vi "Read Refs.vi"(11 "Base Actor in":refnum<class "Base Actor.lvclass">) -> (2 "Refs":refnum<class "Refs.lvclass">)   [LabVIEW 2020, in "jettl.lvlib" / "Base jettl Actor.lvlib" / "Base Actor.lvlib" / "Base Actor.lvclass"]
uses:
  Base Actor.lvclass
  Refs/Refs.lvclass
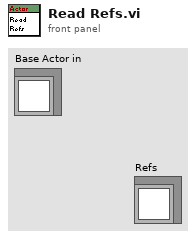
[diagram p1: front panel]
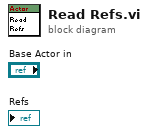
[diagram p0: block diagram]
diagram:
